vi "LabVIEW Year To Version.vi"(0 "LabVIEW Year":u32) -> (2 "LabVIEW Version":string)   [LabVIEW 2019, in "VIPM.lvlib" / "Apply VIPC Step.lvclass"]
uses:
  Apply VIPC Step.lvclass
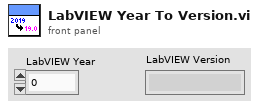
[diagram p1: front panel]
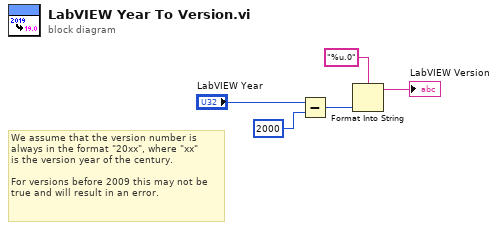
[diagram p0: block diagram]
diagram:
  # "We assume that the version number is\nalways in the format \"20xx\", where \"xx\"\nis the version year of the century.\n\nFor versions before 2009 this may not be\ntrue and will result in an error."
  n1 = Subtract(x="LabVIEW Year", y=u32 2000) -> (x-y=w3:u32)
  n2 = Format Into String(format string="%u.0", w3) -> (resulting string=→"LabVIEW Version":string)  [unwired: 2 in, 1 out]
